vi "Unflatten Value.vi"(8 "error in (no error)":errorcluster, 10 "Value":string, 11 "Boolean in":refnum<class "Assertion 1D.lvclass">) -> (0 "error out":errorcluster, 3 "Boolean out":refnum<class "Assertion 1D.lvclass">)   [LabVIEW 2019, in "Assertion 1D.lvclass"]
uses:
  <vilib>/gpm_packages/@cs/data-type-serializer/source/Assertion 1D/Assertion 1D.lvclass
  <vilib>/gpm_packages/@cs/run-time-assertions/Source/Assert/Assert.lvclass
  <vilib>/gpm_packages/@cs/data-type-serializer/source/Assertion 1D/Assertion 1D.lvclass/Assertion 1D.ctl
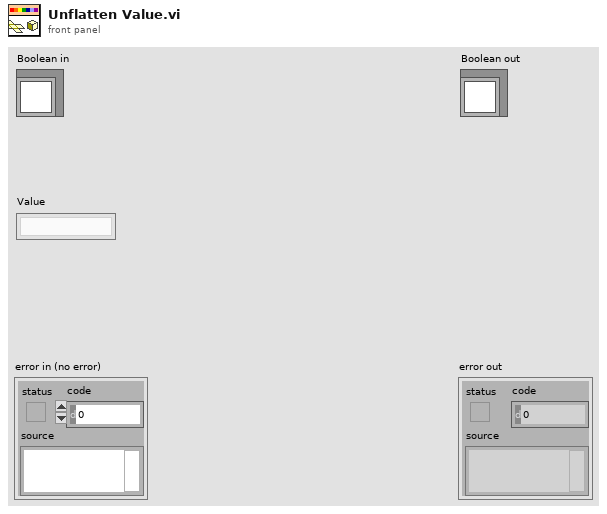
[diagram p1: front panel]
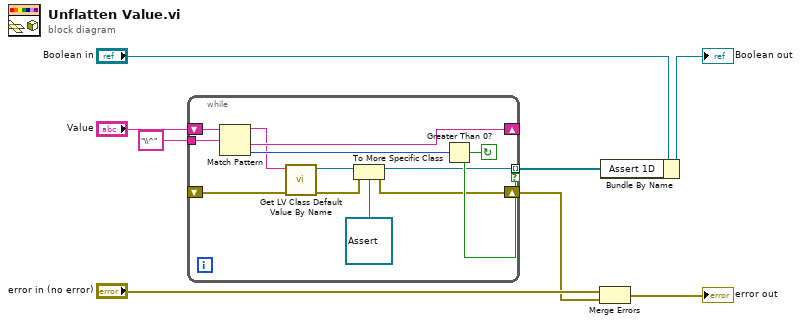
[diagram p0: block diagram]
diagram:
  n1 = while {
    tunnel: "\\^" ("regular expression") -> [w19]
    shift-right: [w18] -> _
    shift-left: "Value" -> [w20]
    tunnel: [w9] -> w2 mode=indexing if=w16
    shift-right: [w10] -> w1
    shift-left: _ -> [w11]
    stop <- w16 continue-if-true
    n2 = Match Pattern(string=w20, regular expression=w19) -> (before substring=w12:string, after substring=w18:string, offset past match=w17:i32)  [unwired: 1 in, 1 out]
    n3 = call <vilib>:"Get LV Class Default Value By Name.vi"("error in (no error)"=w11, "class name"=w12) -> ("error out"=w15:errorcluster, "object"=w14:refnum<class>)  [unwired: 8 in]
    n4 = To More Specific Class(target class=refnum<class "Assert.lvclass"> refnum ("Assert"), reference=w14, error in=w15) -> (specific class reference=w9:refnum<class "Assert.lvclass">, error out=w10:errorcluster)
    n5 = Greater Than 0?(x=w17) -> (x > 0?=w16:bool)
  }
  n6 = Merge Errors("error in (no error)", w1) -> (→"error out":errorcluster)
  n7 = Bundle By Name(cluster="Boolean in", "Assert 1D"=w2) -> (→"Boolean out":refnum<class "Assertion 1D.lvclass">)
